vi "r09543009 劉蓁-太鼓達人.vi"() -> ()   [LabVIEW 2014]
uses:
  <vilib>/sound2/lvsound2.llb/Sound Output Set Volume (Single).vi
panel:
  in  "WindowsMediaPlayer":refnum<k7>(container)
  out "Boolean 3":bool
  out "Boolean 2":bool
  out "Boolean 1":bool
  out "Boolean":bool
  in  "ESC":bool=TRUE
  out "STOP":bool
  out "Score":dbl
  in  "PgDn":bool
  in  "start":bool=TRUE
  in  "PgUP":bool
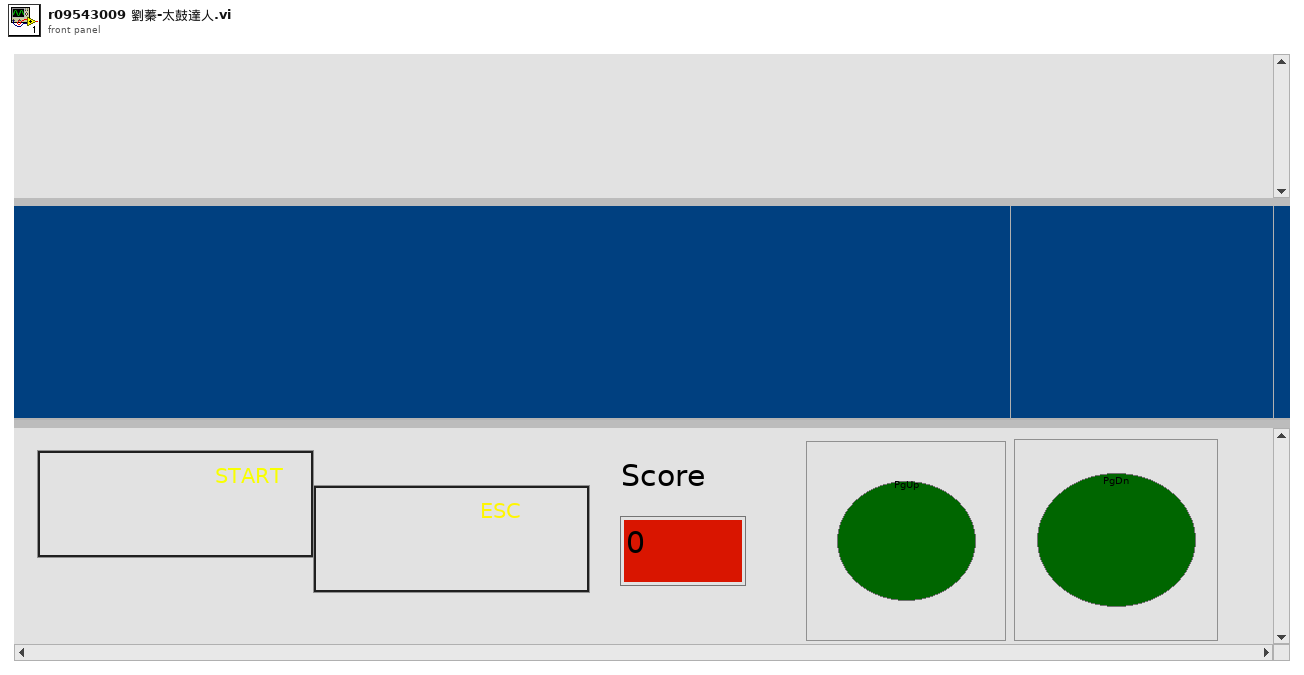
[diagram p1: front panel]
types:
  T1 = typedef "Sound Output Task ID.ctl" = u32
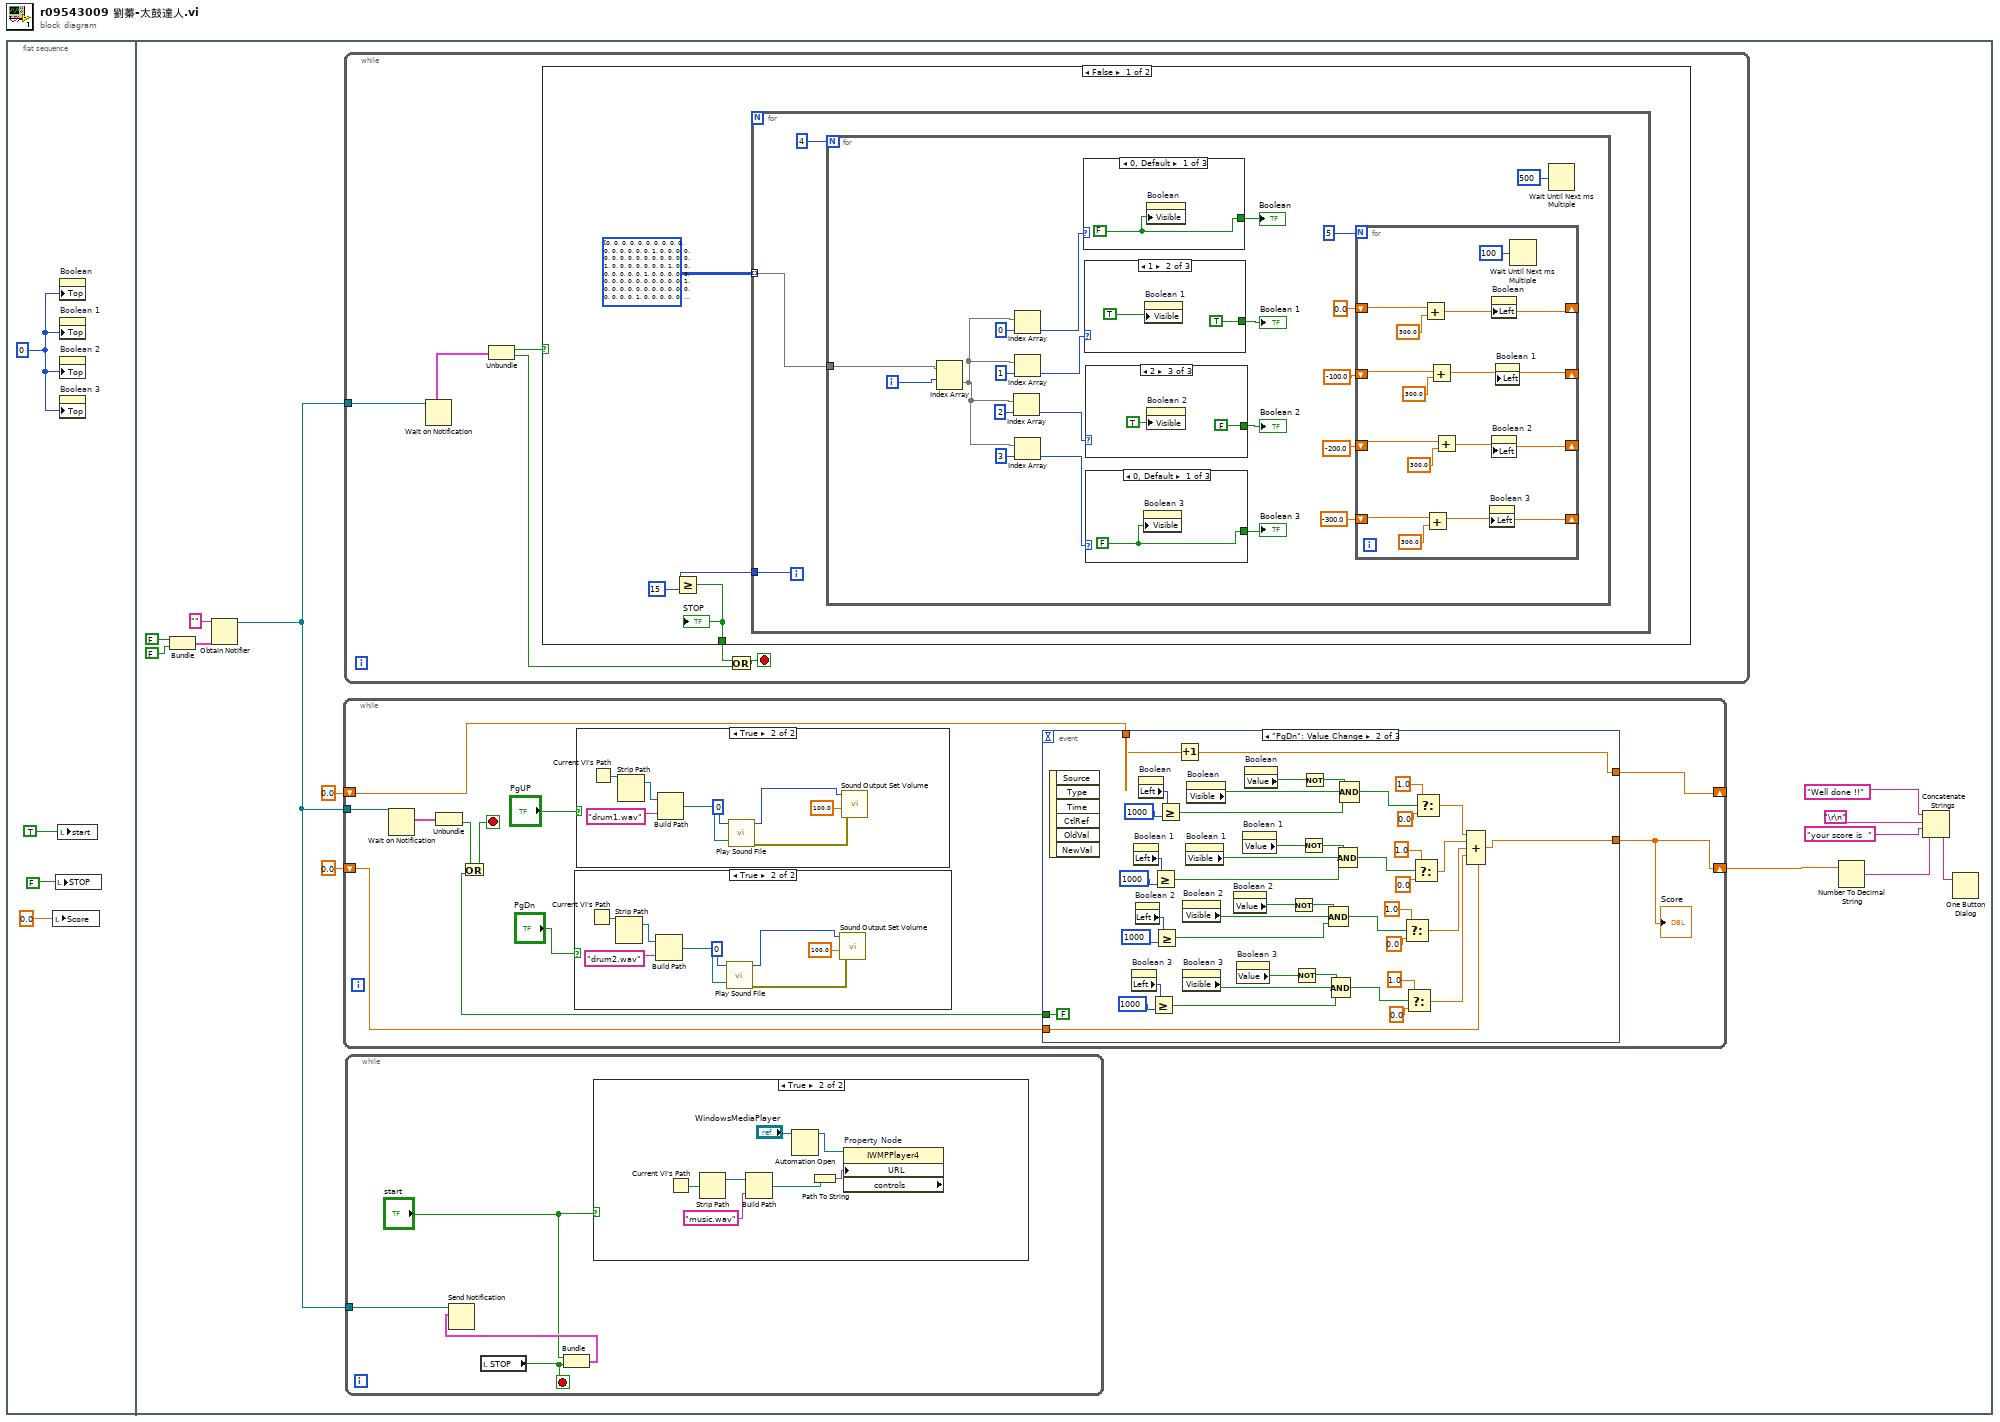
[diagram p0: block diagram]
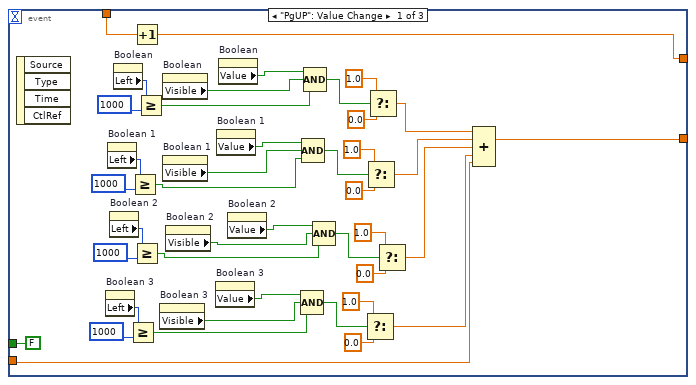
[diagram p4: hidden frame]
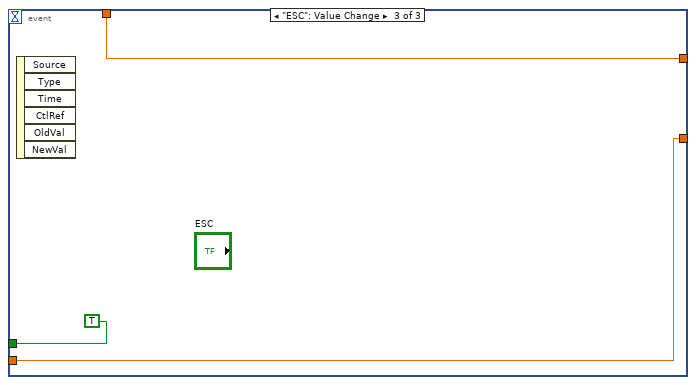
[diagram p5: hidden frame]
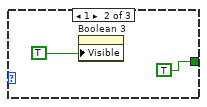
[diagram p7: hidden frame]
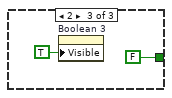
[diagram p8: hidden frame]
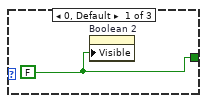
[diagram p9: hidden frame]
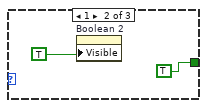
[diagram p10: hidden frame]
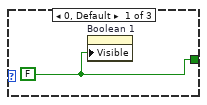
[diagram p11: hidden frame]
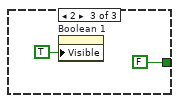
[diagram p12: hidden frame]
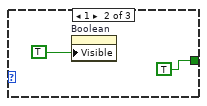
[diagram p13: hidden frame]
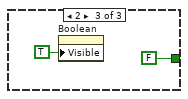
[diagram p14: hidden frame]
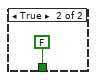
[diagram p15: hidden frame]
diagram:
  n1 = flat-sequence {
    frame #0 {
      w2 = 0 ("Position:Top")
      n2 = local write "Score"(0.0 ("Numeric 2")) -> ()
      n3 = local write "STOP"(FALSE) -> ()
      n4 = local write "start"(TRUE ("OK Button")) -> ()
      n5 = property on="Boolean" class="Bool (strict)"("Top"=w2) -> ()  [unwired: 2 in, 2 out]
      n6 = property on="Boolean 1" class="Bool (strict)"("Top"=w2) -> ()  [unwired: 2 in, 2 out]
      n7 = property on="Boolean 2" class="Bool (strict)"("Top"=w2) -> ()  [unwired: 2 in, 2 out]
      n8 = property on="Boolean 3" class="Bool (strict)"("Top"=w2) -> ()  [unwired: 2 in, 2 out]
    }
    frame #1 {
      n9 = Bundle(FALSE, FALSE) -> (w10:cluster{bool, bool})  [unwired: 1 in]
      n10 = Obtain Notifier(name (unnamed)="", notification data type=w10) -> (notifier out=w7:refnum<notifier>)  [unwired: 2 in, 2 out]
      n11 = while {
        tunnel: w7 -> [w36]
        shift-right: [w35] -> _
        shift-left: 0.0 -> [w37]
        shift-right: [w34] -> w14
        shift-left: 0.0 -> [w33]
        stop <- w29 stop-if-true
        n12 = Wait on Notification(notifier=w36) -> (notification=w39:cluster{bool, bool})  [unwired: 3 in, 3 out]
        n13 = Unbundle(w39) -> (w30:bool)  [unwired: 1 out]
        n14 = case shown="True" "PgDn" {
          frame False {
          }
          frame True {
            n15 = Current VI's Path() -> (path=w45:path)
            n16 = Strip Path(path=w45) -> (stripped path=w44:path)  [unwired: 1 out]
            n17 = Build Path(base path=w44, name or relative path="drum2.wav") -> (appended path=w46:path)
            n18 = call <vilib>:"Play Sound File.vi"("path"=w46, "device ID"=u32 0) -> ("error out"=w41:errorcluster, "task ID"=w42:T1)  [unwired: 8 in]
            n19 = call-poly <vilib>:"Sound Output Set Volume.vi"("error in (no error)"=w41, "volume"=100.0, "task ID"=w42) -> ()  [unwired: 7 in, 2 out]
          }
        }
        n20 = case shown="True" "PgUP" {
          frame False {
          }
          frame True {
            n21 = Current VI's Path() -> (path=w142:path)
            n22 = Strip Path(path=w142) -> (stripped path=w141:path)  [unwired: 1 out]
            n23 = Build Path(base path=w141, name or relative path="drum1.wav") -> (appended path=w143:path)
            n24 = call <vilib>:"Play Sound File.vi"("path"=w143, "device ID"=u32 0) -> ("error out"=w138:errorcluster, "task ID"=w139:T1)  [unwired: 8 in]
            n25 = call-poly <vilib>:"Sound Output Set Volume.vi"("error in (no error)"=w138, "volume"=100.0, "task ID"=w139) -> ()  [unwired: 7 in, 2 out]
          }
        }
        n26 = event shown="[1] \"PgDn\": Value Change" {
          selector: _ -> [_ _ _]
          dyn-events: _ -> [_ _ _]
          timeout: _ -> [_ _ _]
          tunnel: w37 -> [w88 w125 w136]
          tunnel: [w74 w122 w136] -> w35
          tunnel: [w76 w124 w135] -> w34
          tunnel: w33 -> [w75 w123 w135]
          tunnel: [FALSE FALSE TRUE] -> w31
          event "PgUP": Value Change {
            n27 = event-data() -> ()  [unwired: 1 in, 4 out]
            n28 = property on="Boolean 3" class="Bool (strict)"() -> ("Left"=w79:i32)  [unwired: 2 in, 2 out]
            n29 = property on="Boolean 1" class="Bool (strict)"() -> ("Left"=w83:i32)  [unwired: 2 in, 2 out]
            n30 = property on="Boolean 2" class="Bool (strict)"() -> ("Left"=w81:i32)  [unwired: 2 in, 2 out]
            n31 = property on="Boolean" class="Bool (strict)"() -> ("Left"=w87:i32)  [unwired: 2 in, 2 out]
            n32 = Greater Or Equal?(x=w79, y=1000) -> (x >= y?=w52:bool)
            n33 = Greater Or Equal?(x=w83, y=1000) -> (x >= y?=w56:bool)
            n34 = Increment(x=w88) -> (x+1=w74:dbl)
            n35 = Greater Or Equal?(x=w81, y=1000) -> (x >= y?=w54:bool)
            n36 = Greater Or Equal?(x=w87, y=1000) -> (x >= y?=w71:bool)
            n37 = property on="Boolean 3" class="Bool (strict)"() -> ("Visible"=w53:bool)  [unwired: 2 in, 2 out]
            n38 = property on="Boolean" class="Bool (strict)"() -> ("Visible"=w72:bool)  [unwired: 2 in, 2 out]
            n39 = property on="Boolean 1" class="Bool (strict)"() -> ("Visible"=w57:bool)  [unwired: 2 in, 2 out]
            n40 = property on="Boolean 2" class="Bool (strict)"() -> ("Visible"=w55:bool)  [unwired: 2 in, 2 out]
            n41 = property on="Boolean 3" class="Bool (strict)"() -> ("Value"=w59:bool)  [unwired: 2 in, 2 out]
            n42 = property on="Boolean 1" class="Bool (strict)"() -> ("Value"=w67:bool)  [unwired: 2 in, 2 out]
            n43 = property on="Boolean" class="Bool (strict)"() -> ("Value"=w73:bool)  [unwired: 2 in, 2 out]
            n44 = property on="Boolean 2" class="Bool (strict)"() -> ("Value"=w63:bool)  [unwired: 2 in, 2 out]
            n45 = Compound Arithmetic op=AND(w59, w53, w52) -> (w58:bool)
            n46 = Compound Arithmetic op=AND(w67, w57, w56) -> (w66:bool)
            n47 = Compound Arithmetic op=AND(w73, w72, w71) -> (w70:bool)
            n48 = Compound Arithmetic op=AND(w63, w55, w54) -> (w62:bool)
            n49 = Select(t=1.0, s=w58, f=0.0) -> (s? t:f=w49:dbl)
            n50 = Select(t=1.0, s=w66, f=0.0) -> (s? t:f=w51:dbl)
            n51 = Select(t=1.0, s=w70, f=0.0) -> (s? t:f=w77:dbl)
            n52 = Select(t=1.0, s=w62, f=0.0) -> (s? t:f=w50:dbl)
            n53 = Compound Arithmetic op=ADD(w77, w51, w50, w49, w75) -> (w76:dbl)
          }
          event "PgDn": Value Change {
            n54 = event-data() -> ()  [unwired: 1 in, 6 out]
            n55 = property on="Boolean 3" class="Bool (strict)"() -> ("Left"=w132:i32)  [unwired: 2 in, 2 out]
            n56 = property on="Boolean 1" class="Bool (strict)"() -> ("Left"=w128:i32)  [unwired: 2 in, 2 out]
            n57 = property on="Boolean 2" class="Bool (strict)"() -> ("Left"=w130:i32)  [unwired: 2 in, 2 out]
            n58 = property on="Boolean" class="Bool (strict)"() -> ("Left"=w126:i32)  [unwired: 2 in, 2 out]
            n59 = Greater Or Equal?(x=w132, y=1000) -> (x >= y?=w98:bool)
            n60 = Greater Or Equal?(x=w128, y=1000) -> (x >= y?=w102:bool)
            n61 = Greater Or Equal?(x=w130, y=1000) -> (x >= y?=w100:bool)
            n62 = Greater Or Equal?(x=w126, y=1000) -> (x >= y?=w117:bool)
            n63 = Increment(x=w125) -> (x+1=w122:dbl)
            n64 = property on="Boolean 2" class="Bool (strict)"() -> ("Visible"=w101:bool)  [unwired: 2 in, 2 out]
            n65 = property on="Boolean 3" class="Bool (strict)"() -> ("Visible"=w99:bool)  [unwired: 2 in, 2 out]
            n66 = property on="Boolean 1" class="Bool (strict)"() -> ("Visible"=w103:bool)  [unwired: 2 in, 2 out]
            n67 = property on="Boolean" class="Bool (strict)"() -> ("Visible"=w118:bool)  [unwired: 2 in, 2 out]
            n68 = property on="Boolean 2" class="Bool (strict)"() -> ("Value"=w110:bool)  [unwired: 2 in, 2 out]
            n69 = property on="Boolean 3" class="Bool (strict)"() -> ("Value"=w106:bool)  [unwired: 2 in, 2 out]
            n70 = property on="Boolean 1" class="Bool (strict)"() -> ("Value"=w114:bool)  [unwired: 2 in, 2 out]
            n71 = property on="Boolean" class="Bool (strict)"() -> ("Value"=w120:bool)  [unwired: 2 in, 2 out]
            n72 = Not(x=w110) -> (.not. x?=w109:bool)
            n73 = Not(x=w106) -> (.not. x?=w105:bool)
            n74 = Not(x=w114) -> (.not. x?=w113:bool)
            n75 = Not(x=w120) -> (.not. x?=w119:bool)
            n76 = Compound Arithmetic op=AND(w109, w101, w100) -> (w108:bool)
            n77 = Compound Arithmetic op=AND(w105, w99, w98) -> (w104:bool)
            n78 = Compound Arithmetic op=AND(w113, w103, w102) -> (w112:bool)
            n79 = Compound Arithmetic op=AND(w119, w118, w117) -> (w116:bool)
            n80 = Select(t=1.0, s=w108, f=0.0) -> (s? t:f=w95:dbl)
            n81 = Select(t=1.0, s=w104, f=0.0) -> (s? t:f=w94:dbl)
            n82 = Select(t=1.0, s=w112, f=0.0) -> (s? t:f=w96:dbl)
            n83 = Select(t=1.0, s=w116, f=0.0) -> (s? t:f=w97:dbl)
            n84 = Compound Arithmetic op=ADD(w97, w96, w95, w94, w123) -> (w124:dbl)
          }
          event "ESC": Value Change {
            n85 = event-data() -> ()  [unwired: 1 in, 6 out]
          }
        }
        "Score" <- w34
        n86 = Or(x=w30, y=w31) -> (x .or. y?=w29:bool)
      }
      n87 = while {
        tunnel: w7 -> [w146]
        stop <- w145 stop-if-true
        n88 = Wait on Notification(notifier=w146) -> (notification=w150:cluster{bool, bool})  [unwired: 3 in, 3 out]
        n89 = Unbundle(w150) -> (w149:bool, w147:bool)
        n90 = case shown="False" w149 {
          tunnel: [w152 FALSE] -> w148
          frame False {
            n91 = for {
              tunnel: i32[][][] [[[0, 0, 0, 0], [0, 0, 0, 0], [0, 0, 0, 0], [0, 0, 0, 0]], [[1, 0, 0, 0], [0, 0, 0, 0], [0, 0, 0, 0], [0, 0, 0, 0]], [[1, 0, 0, 0], [0, 0, 0, 0], [1, 0, 0, 0], [0, 0, 0, 0]], [[1, 0, 0, 0], [0, 0, 0, 0], [0, 0, 0, 0], [0, 0, 0, 0]], [[1, 0, 0, 0], [0, 0, 0, 0], [0, 0, 0, 0], [0, 0, 0, 0]], [[1, 0, 0, 0], [0, 0, 0, 0], [1, 0, 0, 0], [0, 0, 0, 0]], [[1, 0, 0, 0], [0, 0, 0, 0], [1, 0, 0, 0], [1, 0, 0, 0]], [[1, 0, 0, 0], [0, 0, 0, 0], [1, 0, 0, 0], [0, 0, 0, 0]], [[1, 0, 0, 0], [0, 0, 0, 0], [0, 0, 0, 0], [0, 0, 0, 0]], [[1, 0, 0, 0], [0, 0, 0, 0], [0, 0, 0, 0], [0, 0, 0, 0]], [[1, 0, 0, 0], [0, 0, 0, 0], [0, 0, 0, 0], [0, 0, 0, 0]], [[0, 0, 0, 0], [0, 0, 0, 0], [0, 0, 0, 0], [0, 0, 0, 0]], [[1, 1, 1, 0], [1, 1, 1, 0], [1, 1, 1, 0], [2, 2, 2, 0]], [[1, 1, 1, 0], [1, 1, 1, 0], [1, 1, 1, 0], [2, 2, 2, 0]], [[1, 1, 1, 0], [1, 1, 1, 0], [1, 1, 1, 0], [2, 2, 2, 0]], [[1, 1, 1, 0], [1, 1, 1, 0], [1, 0, 0, 1], [0, 1, 0, 1]], [[0, 0, 0, 0], [0, 0, 0, 0], [0, 0, 0, 0], [0, 0, 0, 0]]] -> [w157] mode=indexing
              tunnel: [w155] -> w151
              i -> [w155]
              n92 = for {
                N: 4 -> [_]
                tunnel: w157 -> [w169]
                i -> [w168]
                n93 = Index Array(array=w169, index (row)=w168) -> (element=w167:i32[])  [unwired: 1 in]
                n94 = Index Array(array=w167, index=2 ("index (row)")) -> (element=w158:i32)
                n95 = Index Array(array=w167, index=0 ("index (row)")) -> (element=w161:i32)
                n96 = Index Array(array=w167, index=1 ("index (row)")) -> (element=w160:i32)
                n97 = Index Array(array=w167, index=3 ("index (row)")) -> (element=w159:i32)
                n98 = case shown="0, Default" w161 {
                  tunnel: [w207 TRUE FALSE] -> w177
                  frame 0, Default {
                    w207 = FALSE ("Visible")
                    n99 = property on="Boolean" class="Bool (strict)"("Visible"=w207) -> ()  [unwired: 2 in, 2 out]
                  }
                  frame 1 {
                    n100 = property on="Boolean" class="Bool (strict)"("Visible"=TRUE) -> ()  [unwired: 2 in, 2 out]
                  }
                  frame 2 {
                    n101 = property on="Boolean" class="Bool (strict)"("Visible"=TRUE) -> ()  [unwired: 2 in, 2 out]
                  }
                }
                "Boolean" <- w177
                n102 = case shown="1" w160 {
                  tunnel: [w202 TRUE FALSE] -> w176
                  frame 0, Default {
                    w202 = FALSE ("Visible")
                    n103 = property on="Boolean 1" class="Bool (strict)"("Visible"=w202) -> ()  [unwired: 2 in, 2 out]
                  }
                  frame 1 {
                    n104 = property on="Boolean 1" class="Bool (strict)"("Visible"=TRUE) -> ()  [unwired: 2 in, 2 out]
                  }
                  frame 2 {
                    n105 = property on="Boolean 1" class="Bool (strict)"("Visible"=TRUE) -> ()  [unwired: 2 in, 2 out]
                  }
                }
                "Boolean 1" <- w176
                n106 = case shown="2" w158 {
                  tunnel: [w197 TRUE FALSE] -> w175
                  frame 0, Default {
                    w197 = FALSE ("Visible")
                    n107 = property on="Boolean 2" class="Bool (strict)"("Visible"=w197) -> ()  [unwired: 2 in, 2 out]
                  }
                  frame 1 {
                    n108 = property on="Boolean 2" class="Bool (strict)"("Visible"=TRUE) -> ()  [unwired: 2 in, 2 out]
                  }
                  frame 2 {
                    n109 = property on="Boolean 2" class="Bool (strict)"("Visible"=TRUE) -> ()  [unwired: 2 in, 2 out]
                  }
                }
                "Boolean 2" <- w175
                n110 = case shown="0, Default" w159 {
                  tunnel: [w192 TRUE FALSE] -> w174
                  frame 0, Default {
                    w192 = FALSE ("Visible")
                    n111 = property on="Boolean 3" class="Bool (strict)"("Visible"=w192) -> ()  [unwired: 2 in, 2 out]
                  }
                  frame 1 {
                    n112 = property on="Boolean 3" class="Bool (strict)"("Visible"=TRUE) -> ()  [unwired: 2 in, 2 out]
                  }
                  frame 2 {
                    n113 = property on="Boolean 3" class="Bool (strict)"("Visible"=TRUE) -> ()  [unwired: 2 in, 2 out]
                  }
                }
                "Boolean 3" <- w174
                n114 = for {
                  N: 5 -> [_]
                  shift-right: [w186] -> _
                  shift-left: 0.0 -> [w187]
                  shift-right: [w184] -> _
                  shift-left: -100.0 -> [w183]
                  shift-right: [w182] -> _
                  shift-left: -200.0 -> [w181]
                  shift-right: [w180] -> _
                  shift-left: -300.0 -> [w179]
                  n115 = Add(x=w187, y=300.0) -> (x+y=w186:dbl)
                  n116 = Add(x=w179, y=300.0) -> (x+y=w180:dbl)
                  n117 = Add(x=w183, y=300.0) -> (x+y=w184:dbl)
                  n118 = Add(x=w181, y=300.0) -> (x+y=w182:dbl)
                  n119 = property on="Boolean 3" class="Bool (strict)"("Left"=w180) -> ()  [unwired: 2 in, 2 out]
                  n120 = property on="Boolean" class="Bool (strict)"("Left"=w186) -> ()  [unwired: 2 in, 2 out]
                  n121 = property on="Boolean 2" class="Bool (strict)"("Left"=w182) -> ()  [unwired: 2 in, 2 out]
                  n122 = property on="Boolean 1" class="Bool (strict)"("Left"=w184) -> ()  [unwired: 2 in, 2 out]
                  n123 = Wait Until Next ms Multiple(millisecond multiple=u32 100) -> ()  [unwired: 1 out]
                }
                n124 = Wait Until Next ms Multiple(millisecond multiple=u32 500) -> ()  [unwired: 1 out]
              }
            }
            n125 = Greater Or Equal?(x=w151, y=15) -> (x >= y?=w152:bool)
            "STOP" <- w152
          }
          frame True {
          }
        }
        n126 = Or(x=w148, y=w147) -> (x .or. y?=w145:bool)
      }
      n127 = while {
        tunnel: w7 -> [w21]
        stop <- w18 stop-if-true
        n128 = local read "STOP"() -> (w18:bool)
        n129 = Bundle("start"="start", "STOP"=w18) -> (w20:cluster{"start":bool, "STOP":bool})  [unwired: 1 in]
        n130 = Send Notification(notification=w20, notifier=w21) -> ()  [unwired: 1 in, 2 out]
        n131 = case shown="True" "start" {
          frame False {
          }
          frame True {
            n132 = Current VI's Path() -> (path=w26:path)
            n133 = Strip Path(path=w26) -> (stripped path=w25:path)  [unwired: 1 out]
            n134 = Build Path(base path=w25, name or relative path="music.wav") -> (appended path=w23:path)
            n135 = Automation Open(Automation Refnum="WindowsMediaPlayer") -> (Automation Refnum=w28:refnum<k7>)  [unwired: 1 in, 3 out]
            n136 = Path To String(path=w23) -> (string=w22:string)
            n137 = property on="Property Node" class="IWMPPlayer4" props=["URL", "controls"](reference=w28, "URL"=w22) -> ()  [unwired: 1 in, 3 out]
          }
        }
      }
      n138 = Number To Decimal String(number=w14) -> (decimal integer string=w13:string)  [unwired: 1 in]
      n139 = Concatenate Strings("Well done !!" ("message"), "\r\n", "your score is  " ("message"), w13) -> (w12:string)
      n140 = One Button Dialog(message=w12) -> ()  [unwired: 1 in, 1 out]
    }
  }
